vi "COM EvolutionBoard.vi"(8 "error in (no error)":errorcluster, 11 "VISA resource name 2":refnum<visa-resource-name>) -> (0 "error out":errorcluster, 2 ".not. x?":bool, 3 "VISA resource name out":refnum<visa-resource-name>)   [LabVIEW 2017]
uses:
  <vilib>/Instr/_visa.llb/VISA Configure Serial Port (Instr).vi
panel:
  in  "Blank Button":bool
  in  "VISA resource name":refnum<visa-resource-name>
  # "Please choose a COM Port of the Evolution Board"
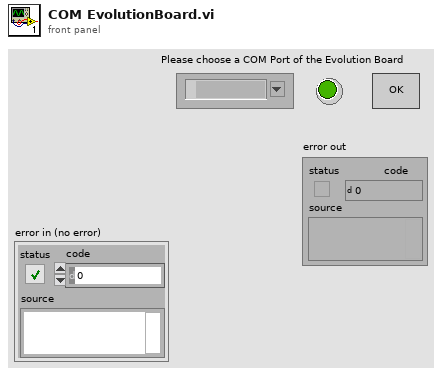
[diagram p1: front panel]
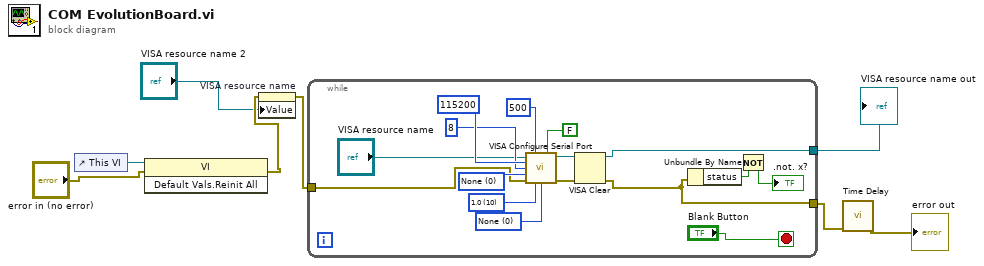
[diagram p0: block diagram]
diagram:
  n1 = control-ref of="This VI"() -> (w6:refnum<vi>)
  n2 = invoke class="VI" method="Default Vals.Reinit All"(reference=w6, error in="error in (no error)") -> (error out=w4:errorcluster)  [unwired: 1 in, 2 out]
  n3 = property on="VISA resource name" class="VISAName"(error in=w4, "Value"="VISA resource name 2") -> (error out=w3:errorcluster)  [unwired: 1 in, 1 out]
  n4 = while {
    tunnel: w3 -> [w11]
    tunnel: [w9] -> w8
    tunnel: [w12] -> w7
    stop <- "Blank Button" stop-if-true
    w17 = u16 0 items=["None"=0, "XON/XOFF"=1, "RTS/CTS"=2, "DTR/DSR"=4] ("flow control")
    w18 = u16 10 items=["1.0"=10, "1.5"=15, "2.0"=20] ("stop bits")
    w19 = u16 0 items=["None", "Odd", "Even", "Mark", "Space"] ("parity")
    n5 = call-poly "VISA Configure Serial Port"("VISA resource name"="VISA resource name", "timeout (10sec)"=u32 500, "Enable Termination\nChar (T)"=FALSE ("Enable Termination\nChar (T)"), "baud rate (9600)"=u32 115200 ("baud rate"), "data bits (8)"=u16 8 ("data bits"), "parity (0:none)"=w19, "error in (no error)"=w11, "stop bits (10: 1 bit)"=w18, "flow control (0:none)"=w17) -> ("VISA resource name out"=w13:refnum<visa-resource-name>, "error out"=w14:errorcluster)  [unwired: 5 in]
    n6 = VISA Clear(VISA resource name=w13, error in (no error)=w14) -> (VISA resource name out=w12:refnum<visa-resource-name>, error out=w9:errorcluster)
    n7 = Unbundle By Name(w9) -> ("status"=w22:bool)
    n8 = Not(x=w22) -> (.not. x?=→".not. x?":bool)
  }
  "VISA resource name out" <- w7
  n9 = call "Time Delay"("error in (no error)"=w8) -> ("error out"=→"error out":errorcluster)  [unwired: 10 in]
